vi "333D01.vi"() -> ()   [LabVIEW 2012]
uses:
  333D Queue Actions.ctl
  <vilib>/Analysis/4window.llb/windowTd.ctl
  <vilib>/sound2/lvsound2.llb/Sound Input Read (DBL).vi
  <vilib>/Analysis/5stat.llb/RMS (DBL).vi
  <vilib>/Analysis/0measdsp.llb/Scaled Time Domain Window (DBL).vi
  <vilib>/Analysis/NI_AALPro.lvlib
panel:
  out "333D01 Information":T1
  out "AvgCounts":u16 caption="/"
  in  "Average Counts":u16=10
  in  "Average":bool
  in  "Sample Rate (Hz)":dbl(ring)=8000.0 items=["8000 Hz"=8000.0, "11025 Hz"=11025.0, "16000 Hz"=16000.0, "22050 Hz"=22050.0, "32000 Hz"=32000.0, "44100 Hz"=44100.0, "48000 Hz"=48000.0]
  in  "Enable Cursor Reading":bool=TRUE
  in  "1st Cursor  to  Max Y":bool=TRUE caption="Harmonic Cursor\nwith 1st Cursor  to  Max Y"
  out "B: Sens (mV/g)":dbl caption="B:"
  out "A: Sens (mV/g)":dbl caption="A:"
  out "B: Overall (mV-rms)":dbl caption="B:" format="%#_4g"
  out "A: Overall (mV-rms)":dbl caption="A:" format="%#_4g"
  out "B: Overall (g-rms)":dbl caption="B:" format="%0.4f"
  out "A: Overall (g-rms)":dbl caption="A:" format="%0.4f"
  out "Cursors":string[][](table)
  in  "Enable Cursors":bool=TRUE
  in  "Window":T2=6 items=["Rectangle"=0, "Hanning"=1, "Hamming"=2, "Blackman-Harris"=3, "Exact Blackman"=4, "Blackman"=5, "Flat Top"=6, "4 Term B-Harris "=7, "7 Term B-Harris"=8, "Low Sidelobe"=9, "Blackman Nuttall"=11, "Triangle"=30, "Bartlett-Hanning"=31, "Bohman"=32, "Parzen"=33, "Welch"=34, "Kaiser"=60, "Dolph-Chebyshev"=61, "Gaussian"=62]
  in  "Aquire":bool=TRUE
  in  "Analyze":bool
  out "String":string
  in  "Queue Actions":T3
  out "B: Max (mV)":dbl
  out "A: Max (mV)":dbl
  in  "Sensitivity B (Counts / m/s^2)":i32=72139 caption="Chan B"
  in  "Sensitivity A (Counts / m/s^2)":i32=37426 caption="Chan A"
  out "Freq (Hz)":dbl
  out "B: Max (g peak)":dbl
  out "Spec":cluster{"Y":dbl[], "Y":dbl[]}[](graph)
  out "max index(es)":i32
  out "A: Max (g peak)":dbl
  out "Windowed":waveform(dbl)[](graph)
  out "data":waveform(dbl)[](array[waveform])
  out "Device Name":string
  in  "Device ID":u32
  out "Time":waveform(dbl)[](graph)
  in  "number of samples/ch":i32=4096
  in  "Quit":bool
  # "Overall (mV-rms):"
  # "Sensitivity (mV/g):"
  # "Overall (g-rms)"
  # "Acquisition Setup"
  # "Sensor Information"
  # "Sensitivity (Counts / m/s^2)"
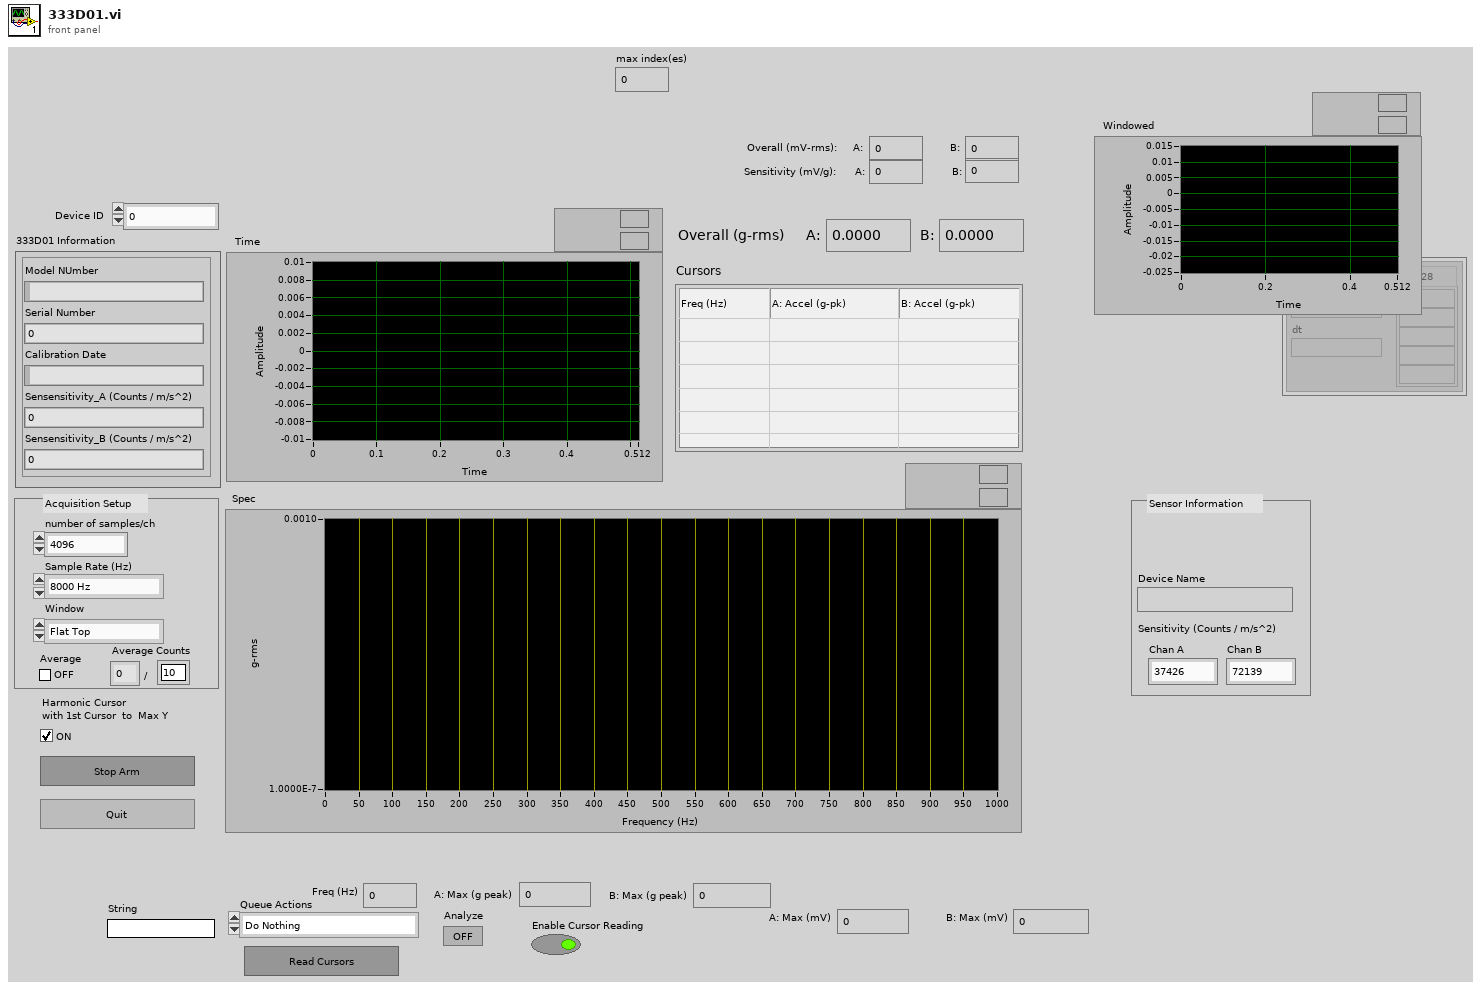
[diagram p1: front panel]
types:
  T1 = cluster{"Model NUmber":string, "Calibration Date":string, "Sensensitivity_A (Counts / m/s^2)":u64, "Sensensitivity_B (Counts / m/s^2)":u64, "Serial Number":u64}
  T2 = typedef "NI_AALPro.lvlib/windowTd.ctl" = u32
  T3 = typedef "333D Queue Actions.ctl" = enum16{"Do Nothing", "Initialize", "Process Data", "Process Cursors", "Pick Cursor", "Return"}
  T4 = cluster{"Model NUmber":string, "Calibration Date":string, "Sensensitivity_A":u64, "Sensensitivity_B":u64, "Serial Number":u64}
  T5 = cluster{"Sample Rate (Hz)":dbl, "Channels":i32, "Bits":i32}
  T6 = typedef "Sound Input Task ID.ctl" = u32
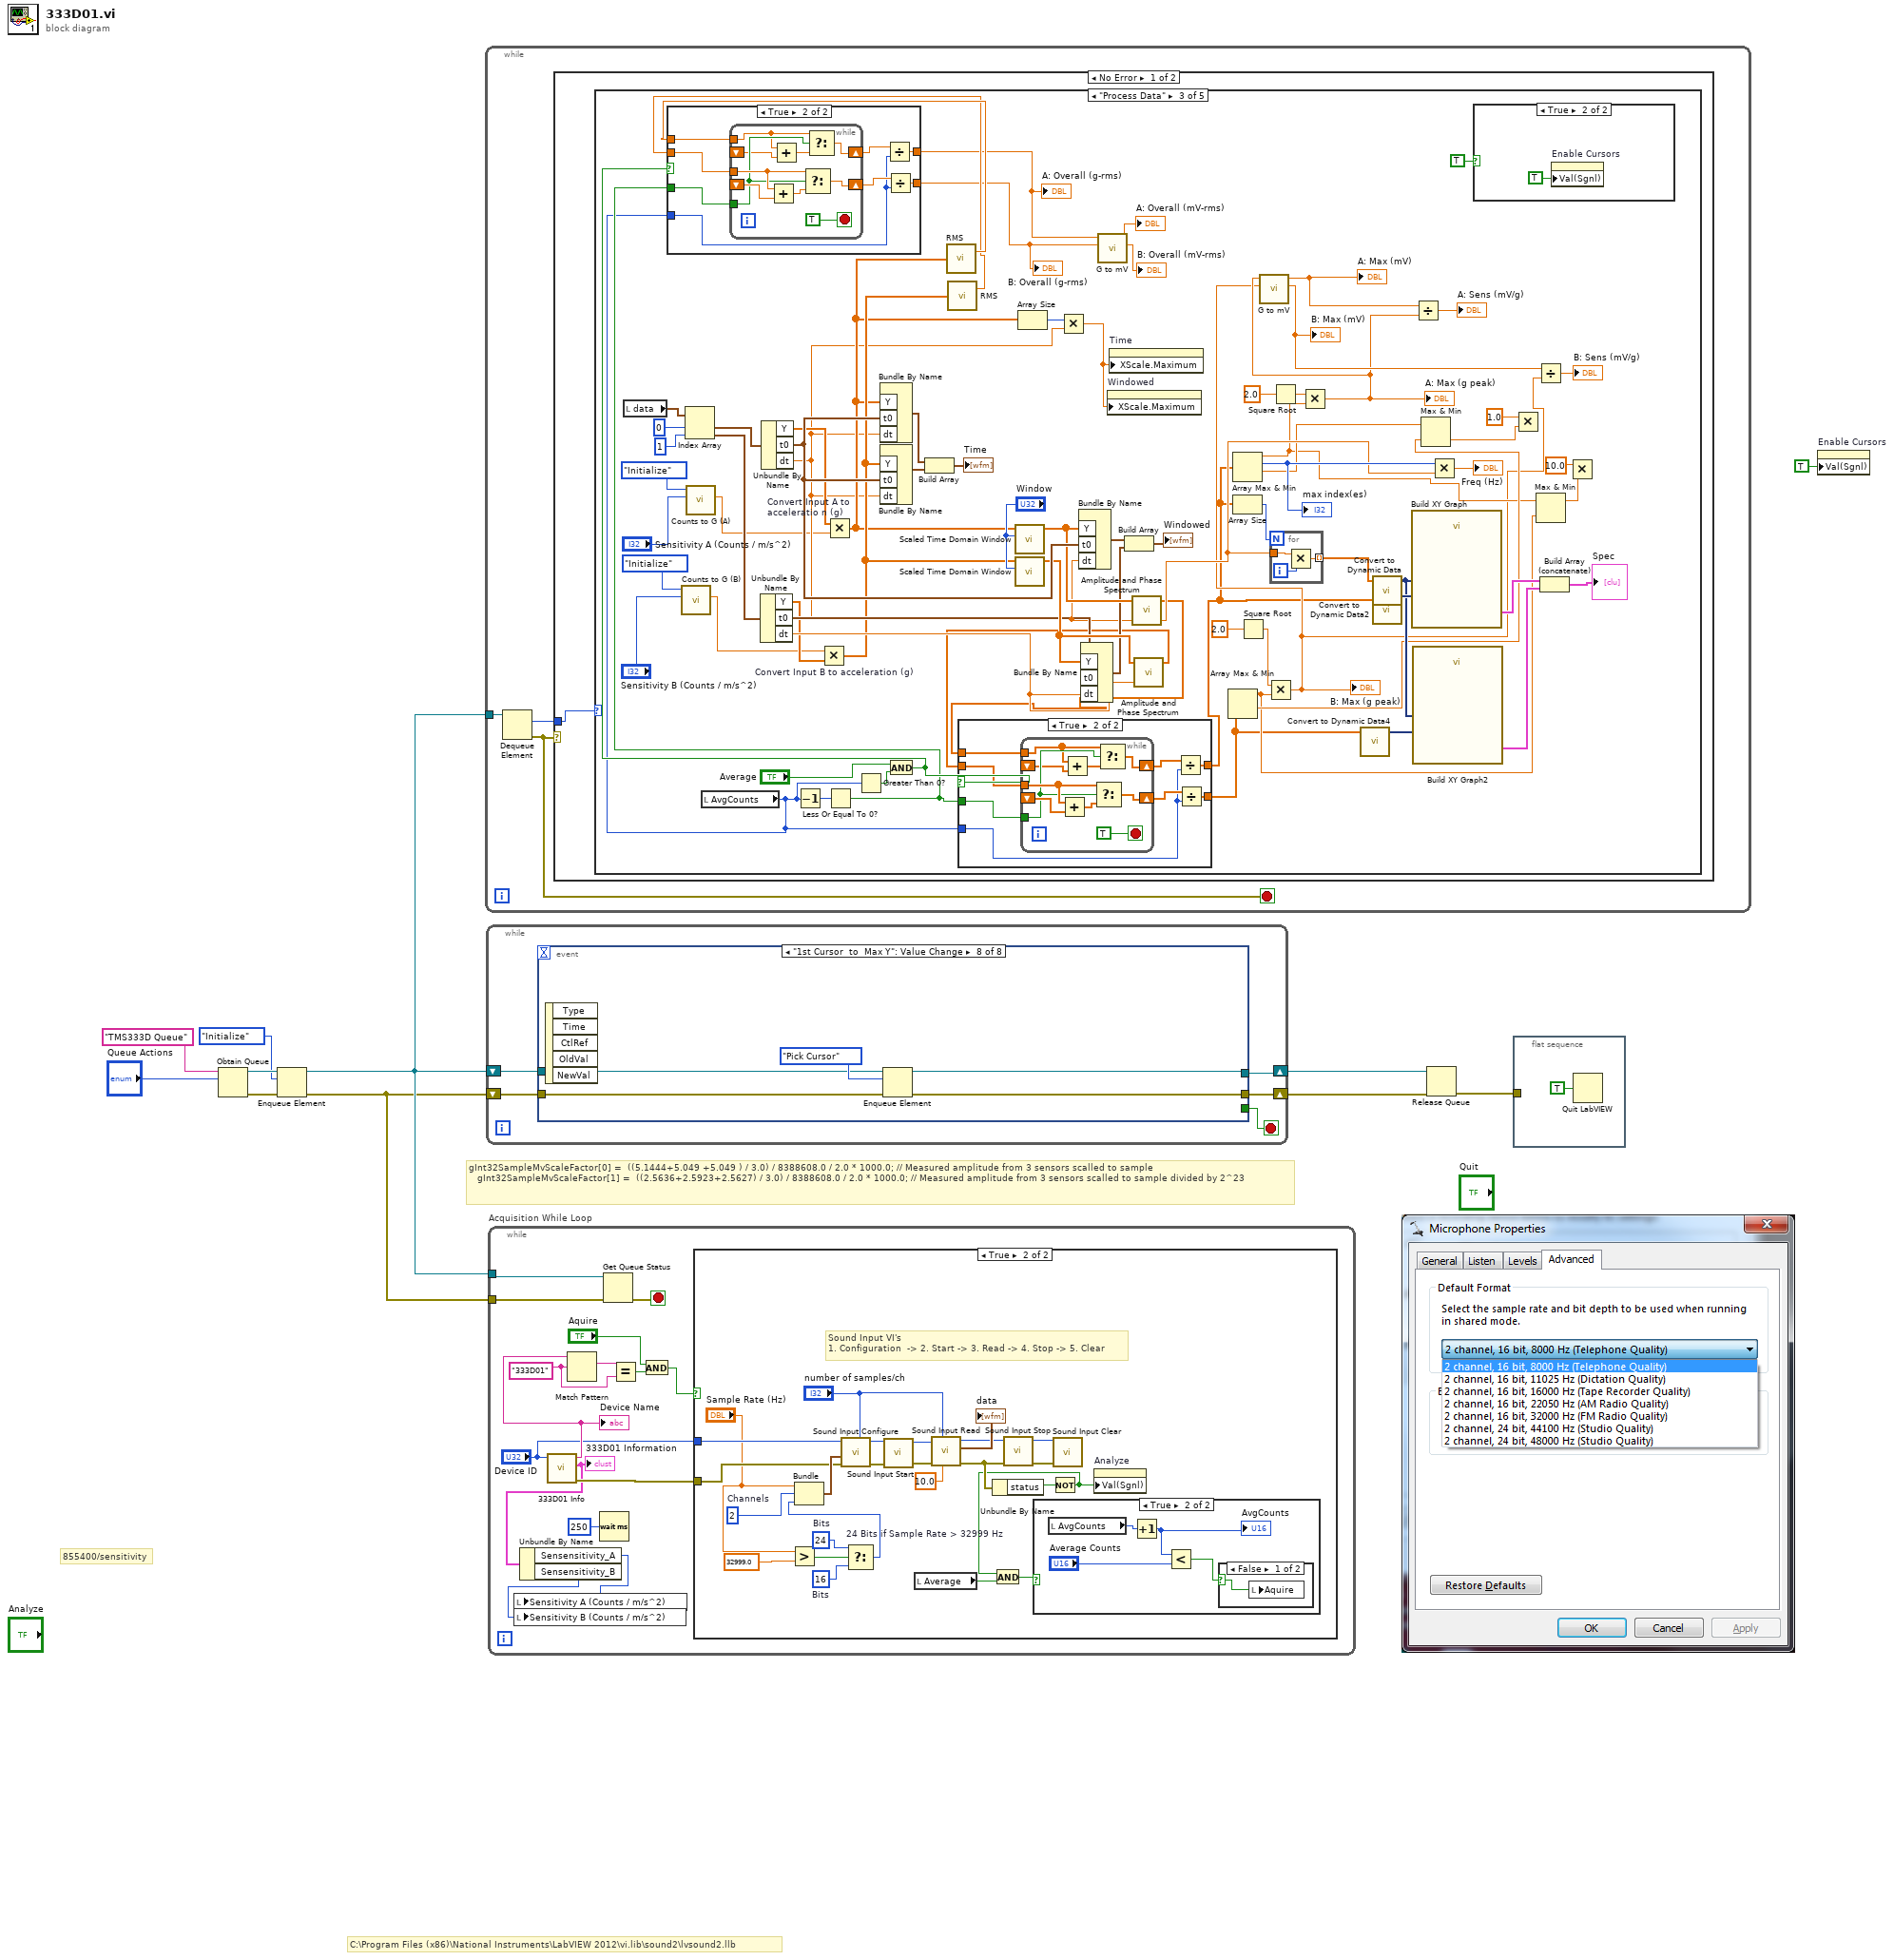
[diagram p0: block diagram]
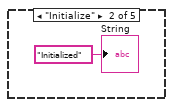
[diagram p6: hidden frame]
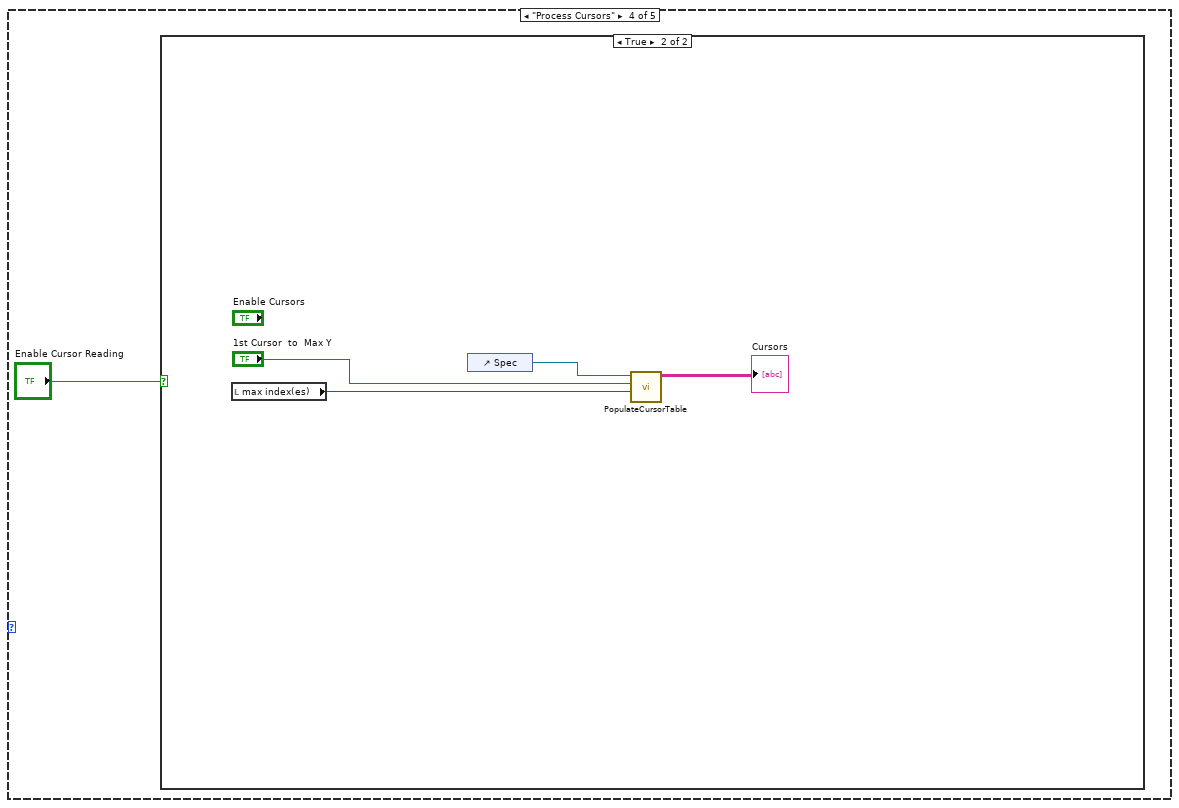
[diagram p10: hidden frame]
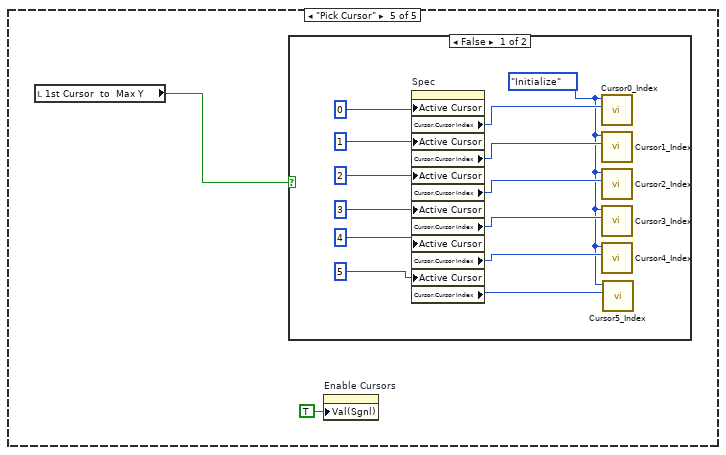
[diagram p12: hidden frame]
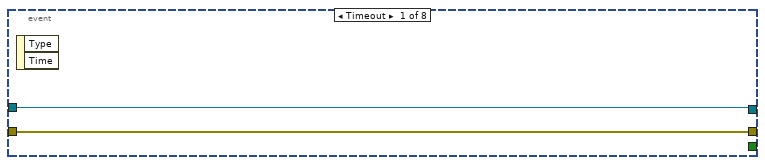
[diagram p15: hidden frame]
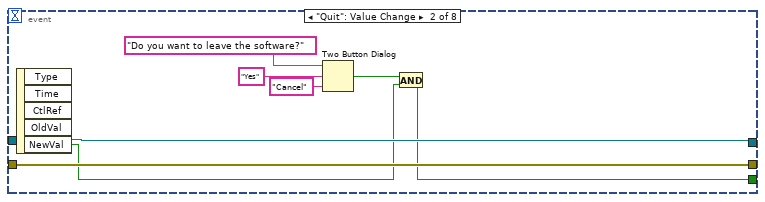
[diagram p16: hidden frame]
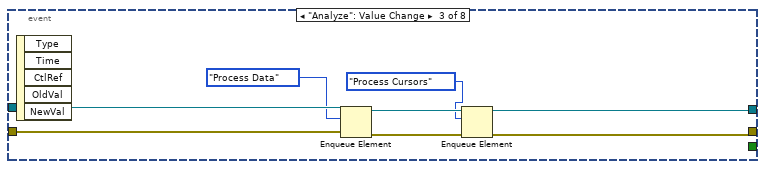
[diagram p17: hidden frame]
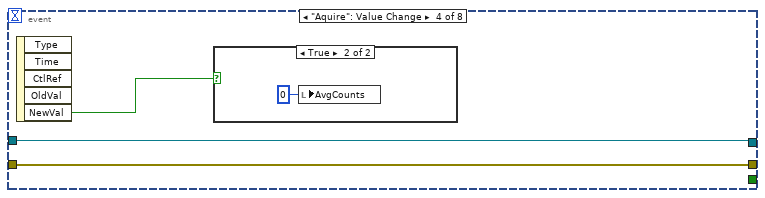
[diagram p18: hidden frame]
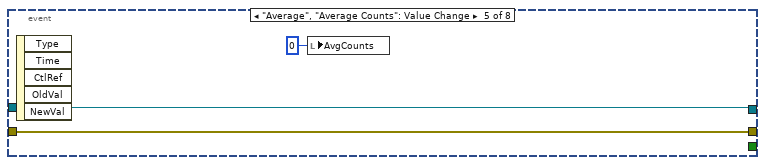
[diagram p20: hidden frame]
diagram:
  # "gInt32SampleMvScaleFactor[0] =  ((5.1444+5.049 +5.049 ) / 3.0) / 8388608.0 / 2.0 * 1000.0; // Measured amplitude from 3 sensors scalled to sample\n\t\t\tgInt32SampleMvScaleFactor[1] =  ((2.5636+2.5923+2.5627) / 3.0) / 8388608.0 / 2.0 * 1000.0; // Measured amplitude from 3 sensors scalled to sample divided by 2^23"
  # "855400/sensitivity"
  # "C:\\Program Files (x86)\\National Instruments\\LabVIEW 2012\\vi.lib\\sound2\\lvsound2.llb"
  n1 = Obtain Queue(name (unnamed)="TMS333D Queue", element data type="Queue Actions") -> (queue out=w9:refnum<queue>, error out=w8:errorcluster)  [unwired: 3 in, 1 out]
  n2 = Enqueue Element(queue=w9, element=333D_Queue_Actions."Initialize" ("Queue Actions"), error in (no error)=w8) -> (queue out=w4:refnum<queue>, error out=w3:errorcluster)  [unwired: 1 in, 1 out]
  n3 = while {
    tunnel: w4 -> [w14]
    stop <- w13 stop-if-true
    n4 = Dequeue Element(queue=w14) -> (element=w12:T3, error out=w13:errorcluster)  [unwired: 2 in, 2 out]
    n5 = case shown="No Error" w13 {
      tunnel: w12 -> [w15 _]
      frame No Error {
        n6 = case shown="\"Process Data\"" w15 {
          frame "Do Nothing", Default {
          }
          frame "Initialize" {
            "String" <- "Initialized" ("String")
          }
          frame "Process Data" {
            n7 = local read "data"() -> (w61:waveform(dbl)[])
            n8 = call "Counts to G (B).vi"("(Counts / m/s^2)"="Sensitivity B (Counts / m/s^2)", "Action"=enum16{"Initialize", "Read"}."Initialize") -> ("OutputB (g)"=w39:dbl)  [unwired: 8 in, 1 out]
            n9 = Index Array(array=w61, index #1=0 ("index"), index #2=1 ("index")) -> (element #1=w63:waveform(dbl), element #2=w66:waveform(dbl))
            n10 = call "Counts to G (A).vi"("(Counts / m/s^2)"="Sensitivity A (Counts / m/s^2)", "Action"=enum16{"Initialize", "Read"}."Initialize") -> ("Output (g)"=w41:dbl)  [unwired: 8 in, 1 out]
            n11 = local read "AvgCounts"() -> (w17:u16)
            n12 = Unbundle By Name(w66) -> ("Y"=w67:dbl[], "t0"=w68:timestamp, "dt"=w73:dbl)
            n13 = Unbundle By Name(w63) -> ("Y"=w89:dbl[], "t0"=w91:timestamp, "dt"=w48:dbl)
            n14 = Decrement(x=w17) -> (x-1=w30:u16)
            n15 = Multiply "Convert Input B to acceleration (g)"(x=w39, y=w67) -> (x*y=w54:dbl[])
            n16 = Multiply "Convert Input A to acceleratio n (g)"(x=w89, y=w41) -> (x*y=w50:dbl[])
            n17 = Less Or Equal To 0?(x=w30) -> (x <= 0?=w20:bool)
            n18 = Greater Than 0?(x=w17) -> (x > 0?=w18:bool)
            n19 = Bundle By Name("Y"=w50, "t0"=w91, "dt"=w48) -> (w88:waveform(dbl))  [unwired: 1 in]
            n20 = Bundle By Name("Y"=w54, "t0"=w91, "dt"=w48) -> (w92:waveform(dbl))  [unwired: 1 in]
            n21 = And(x="Average", y=w18) -> (x .and. y?=w21:bool)
            n22 = Build Array(w88, w92) -> (→"Time":waveform(dbl)[])
            n23 = call-poly <vilib>:"RMS.vi"("X"=w50) -> ("rms value"=w26:dbl)  [unwired: 1 out]
            n24 = call-poly <vilib>:"RMS.vi"("X"=w54) -> ("rms value"=w25:dbl)  [unwired: 1 out]
            n25 = case shown="True" w21 {
              tunnel: w25 -> [w94 w102]
              tunnel: w20 -> [_ w101]
              tunnel: w17 -> [_ w96]
              tunnel: [w94 w99] -> w22
              tunnel: w26 -> [w93 w98]
              tunnel: [w93 w95] -> w23
              frame False {
              }
              frame True {
                n26 = while {
                  shift-right: [w111] -> w100
                  shift-left: _ -> [w109]
                  tunnel: w102 -> [w110]
                  tunnel: w101 -> [w106]
                  tunnel: w98 -> [w105]
                  shift-right: [w107] -> w97
                  shift-left: _ -> [w104]
                  stop <- TRUE stop-if-true
                  n27 = Add(x=w110, y=w109) -> (x+y=w108:dbl)
                  n28 = Add(x=w105, y=w104) -> (x+y=w103:dbl)
                  n29 = Select(t=w110, s=w106, f=w108) -> (s? t:f=w111:dbl)
                  n30 = Select(t=w105, s=w106, f=w103) -> (s? t:f=w107:dbl)
                }
                n31 = Divide(x=w97, y=w96) -> (x/y=w95:dbl)
                n32 = Divide(x=w100, y=w96) -> (x/y=w99:dbl)
              }
            }
            "A: Overall (g-rms)" <- w23
            "B: Overall (g-rms)" <- w22
            n33 = call-poly <vilib>:"Scaled Time Domain Window.vi"("window"="Window", "X"=w50) -> ("Windowed X"=w71:dbl[])  [unwired: 7 in, 2 out]
            n34 = call-poly <vilib>:"Scaled Time Domain Window.vi"("window"="Window", "X"=w54) -> ("Windowed X"=w72:dbl[])  [unwired: 7 in, 2 out]
            n35 = Array Size(array=w50) -> (size(s)=w49:i32)
            n36 = Multiply(x=w49, y=w48) -> (x*y=w47:dbl)
            n37 = Bundle By Name("Y"=w71, "t0"=w91, "dt"=w48) -> (w64:waveform(dbl))  [unwired: 1 in]
            n38 = Bundle By Name("Y"=w72, "t0"=w68, "dt"=w73) -> (w70:waveform(dbl))  [unwired: 1 in]
            n39 = call "G to mV.vi"("Ain (g)"=w22, "Bin (g)"=w23) -> ("B out (mV)"=→"B: Overall (mV-rms)":dbl, "A out (mV)"=→"A: Overall (mV-rms)":dbl)  [unwired: 6 in]
            n40 = property on="Windowed" class="WFGraph (strict)"("XScale.Maximum"=w47) -> ()  [unwired: 2 in, 2 out]
            n41 = property on="Time" class="WFGraph (strict)"("XScale.Maximum"=w47) -> ()  [unwired: 2 in, 2 out]
            n42 = Build Array(w64, w70) -> (→"Windowed":waveform(dbl)[])
            n43 = call <vilib>:"Amplitude and Phase Spectrum.vi"("dt"=w48, "Signal (V)"=w71) -> ("df"=w81:dbl, "Amp Spectrum Mag (Vrms)"=w28:dbl[])  [unwired: 1 in, 1 out]
            n44 = call <vilib>:"Amplitude and Phase Spectrum.vi"("dt"=w73, "Signal (V)"=w72) -> ("Amp Spectrum Mag (Vrms)"=w31:dbl[])  [unwired: 1 in, 2 out]
            n45 = case shown="True" w21 {
              tunnel: w31 -> [w114 w122]
              tunnel: w20 -> [_ w121]
              tunnel: w17 -> [_ w116]
              tunnel: [w114 w119] -> w29
              tunnel: w28 -> [w113 w118]
              tunnel: [w113 w115] -> w27
              frame False {
              }
              frame True {
                n46 = while {
                  shift-right: [w131] -> w120
                  shift-left: _ -> [w129]
                  tunnel: w122 -> [w130]
                  tunnel: w121 -> [w126]
                  tunnel: w118 -> [w125]
                  shift-right: [w127] -> w117
                  shift-left: _ -> [w124]
                  stop <- TRUE stop-if-true
                  n47 = Add(x=w130, y=w129) -> (x+y=w128:dbl[])
                  n48 = Add(x=w125, y=w124) -> (x+y=w123:dbl[])
                  n49 = Select(t=w130, s=w126, f=w128) -> (s? t:f=w131:dbl[])
                  n50 = Select(t=w125, s=w126, f=w123) -> (s? t:f=w127:dbl[])
                }
                n51 = Divide(x=w117, y=w116) -> (x/y=w115:dbl[])
                n52 = Divide(x=w120, y=w116) -> (x/y=w119:dbl[])
              }
            }
            n53 = Array Max & Min(array=w29) -> (max value=w52:dbl, min value=w57:dbl)  [unwired: 2 out]
            n54 = Array Max & Min(array=w27) -> (max value=w53:dbl, max index (indices)=w82:i32, min value=w58:dbl)  [unwired: 1 out]
            "max index(es)" <- w82
            n55 = Array Size(array=w27) -> (size(s)=w74:i32)
            n56 = Square Root(x=2.0) -> (sqrt(x)=w87:dbl)
            n57 = Multiply(x=w87, y=w52) -> (x*y=w35:dbl)
            "B: Max (g peak)" <- w35
            n58 = for {
              N: w74 -> [_]
              tunnel: w81 -> [w135]
              tunnel: [w134] -> w76 mode=indexing
              i -> [w136]
              n59 = Multiply(x=w135, y=w136) -> (x*y=w134:dbl)
            }
            n60 = Square Root(x=2.0) -> (sqrt(x)=w84:dbl)
            n61 = Multiply(x=w84, y=w53) -> (x*y=w36:dbl)
            "A: Max (g peak)" <- w36
            n62 = call "G to mV.vi"("Ain (g)"=w35, "Bin (g)"=w36) -> ("B out (mV)"=w45:dbl, "A out (mV)"=w46:dbl)  [unwired: 6 in]
            "A: Max (mV)" <- w46
            "B: Max (mV)" <- w45
            n63 = call "Convert to Dynamic Data4"("Array"=w29) -> ("Dynamic Data Type"=w75:dynamicdata)  [unwired: 3 in]
            n64 = call "Convert to Dynamic Data"("Array"=w76) -> ("Dynamic Data Type"=w59:dynamicdata)  [unwired: 3 in]
            n65 = call "Convert to Dynamic Data2"("Array"=w27) -> ("Dynamic Data Type"=w77:dynamicdata)  [unwired: 3 in]
            n66 = call "Build XY Graph"("Y Input"=w77, "X Input"=w59) -> ("XY Graph"=w78:cluster{"Y":dbl[], "Y":dbl[]}[])  [unwired: 3 in, 6 out]
            n67 = call "Build XY Graph2"("Y Input"=w75, "X Input"=w59) -> ("XY Graph"=w79:cluster{"Y":dbl[], "Y":dbl[]}[])  [unwired: 3 in, 6 out]
            n68 = Divide(x=w46, y=w36) -> (x/y=→"A: Sens (mV/g)":dbl)
            n69 = Max & Min(x=w58, y=w57) -> (min(x,y)=w56:dbl)  [unwired: 1 out]
            n70 = Multiply(x=w82, y=w81) -> (x*y=→"Freq (Hz)":dbl)
            n71 = case shown="True" TRUE {
              frame False {
              }
              frame True {
                n72 = property on="Enable Cursors" class="Bool (strict)"("Val(Sgnl)"=TRUE ("Value (Signaling)")) -> ()  [unwired: 2 in, 2 out]
              }
            }
            n73 = Multiply(x=1.0, y=w56) -> ()  [unwired: 1 out]
            n74 = Divide(x=w45, y=w35) -> (x/y=→"B: Sens (mV/g)":dbl)
            n75 = Max & Min(x=w53, y=w52) -> (max(x,y)=w51:dbl)  [unwired: 1 out]
            n76 = Build Array (concatenate)(w78, w79) -> (→"Spec":cluster{"Y":dbl[], "Y":dbl[]}[])
            n77 = Multiply(x=10.0, y=w51) -> ()  [unwired: 1 out]
          }
          frame "Process Cursors" {
            n78 = case shown="True" "Enable Cursor Reading" {
              frame False {
              }
              frame True {
                n79 = local read "max index(es)"() -> (w140:i32)
                n80 = control-ref of="Spec"() -> (w138:refnum<vi>)
                n81 = call "PopulateCursorTable.vi"("max index(es)"=w140, "1st Cursor  to  Max Y"="1st Cursor  to  Max Y", "XYGraph in"=w138) -> ("Array"=→"Cursors":string[][])  [unwired: 8 in]
              }
            }
          }
          frame "Pick Cursor" {
            n82 = local read "1st Cursor  to  Max Y"() -> (w143:bool)
            n83 = case shown="False" w143 {
              frame False {
                w145 = enum16{"Initialize", "Read"}."Initialize" ("Action")
                n84 = property on="Spec" class="XYGraph (strict)"("Active Cursor"=u32 0, "Active Cursor"=1 ("Cursor.Cursor Index"), "Active Cursor"=u32 2, "Active Cursor"=u32 3, "Active Cursor"=u32 4, "Active Cursor"=u32 5) -> ("Cursor.Cursor Index"=w151:i32, "Cursor.Cursor Index"=w150:i32, "Cursor.Cursor Index"=w149:i32, "Cursor.Cursor Index"=w148:i32, "Cursor.Cursor Index"=w147:i32, "Cursor.Cursor Index"=w144:i32)  [unwired: 2 in, 2 out]
                n85 = call "Cursor0_Index.vi"("Input"=w151, "Action"=w145) -> ()  [unwired: 8 in, 2 out]
                n86 = call "Cursor1_Index.vi"("Input"=w150, "Action"=w145) -> ()  [unwired: 8 in, 2 out]
                n87 = call "Cursor2_Index.vi"("Input"=w149, "Action"=w145) -> ()  [unwired: 8 in, 2 out]
                n88 = call "Cursor3_Index.vi"("Input"=w148, "Action"=w145) -> ()  [unwired: 8 in, 2 out]
                n89 = call "Cursor4_Index.vi"("Input"=w147, "Action"=w145) -> ()  [unwired: 8 in, 2 out]
                n90 = call "Cursor5_Index.vi"("Input"=w144, "Action"=w145) -> ()  [unwired: 8 in, 2 out]
              }
              frame True {
              }
            }
            n91 = property on="Enable Cursors" class="Bool (strict)"("Val(Sgnl)"=TRUE ("Value (Signaling)")) -> ()  [unwired: 2 in, 2 out]
          }
        }
      }
      frame Error {
      }
    }
  }
  n92 = while {
    shift-right: [w159] -> w6
    shift-left: w4 -> [w161]
    shift-right: [w158] -> w5
    shift-left: w3 -> [w160]
    stop <- w157 stop-if-true
    n93 = event shown="[7] \"1st Cursor  to  Max Y\": Value Change" {
      selector: _ -> [_ _ _ _ _ _ _ _]
      dyn-events: _ -> [_ _ _ _ _ _ _ _]
      timeout: _ -> [_ _ _ _ _ _ _ _]
      tunnel: [w163 w171 w175 w182 w186 w190 w200 w205] -> w159
      tunnel: w161 -> [w163 w171 w179 w182 w186 w191 w202 w207]
      tunnel: w160 -> [w162 w170 w178 w181 w185 w189 w201 w206]
      tunnel: [w162 w170 w173 w181 w185 w188 w199 w204] -> w158
      tunnel: [_ w164 _ _ _ _ _ _] -> w157
      event Timeout {
        n94 = event-data() -> ()  [unwired: 1 in, 2 out]
      }
      event "Quit": Value Change {
        n95 = event-data() -> ("NewVal"=w165:bool)  [unwired: 1 in, 4 out]
        n96 = Two Button Dialog(message="Do you want to leave the software?", 1:"Cancel" ("F button name (\"Cancel\")"), 2:"Yes" ("T button name (\"OK\")")) -> (T button?=w166:bool)
        n97 = And(x=w166, y=w165) -> (x .and. y?=w164:bool)
      }
      event "Analyze": Value Change {
        n98 = event-data() -> ()  [unwired: 1 in, 5 out]
        n99 = Enqueue Element(queue=w179, element=333D_Queue_Actions."Process Data", error in (no error)=w178) -> (queue out=w176:refnum<queue>, error out=w174:errorcluster)  [unwired: 1 in, 1 out]
        n100 = Enqueue Element(queue=w176, element=333D_Queue_Actions."Process Cursors", error in (no error)=w174) -> (queue out=w175:refnum<queue>, error out=w173:errorcluster)  [unwired: 1 in, 1 out]
      }
      event "Aquire": Value Change {
        n101 = event-data() -> ("NewVal"=w180:bool)  [unwired: 1 in, 4 out]
        n102 = case shown="True" w180 {
          frame False {
          }
          frame True {
            n103 = local write "AvgCounts"(u16 0 ("AvgCounts")) -> ()
          }
        }
      }
      event "Average", "Average Counts": Value Change {
        n104 = event-data() -> ()  [unwired: 1 in, 5 out]
        n105 = local write "AvgCounts"(u16 0 ("AvgCounts")) -> ()
      }
      event "Enable Cursors": Value Change {
        n106 = event-data() -> ()  [unwired: 1 in, 5 out]
        n107 = case shown="True" TRUE {
          tunnel: w191 -> [w193 w198]
          tunnel: [w193 w197] -> w190
          tunnel: w189 -> [w192 w196]
          tunnel: [w192 w195] -> w188
          frame False {
          }
          frame True {
            n108 = Enqueue Element(queue=w198, element=333D_Queue_Actions."Process Cursors", error in (no error)=w196) -> (queue out=w197:refnum<queue>, error out=w195:errorcluster)  [unwired: 1 in, 1 out]
          }
        }
      }
      event "Spec": Cursor Move; "Spec": Cursor Grab; "Spec": Cursor Release {
        n109 = event-data() -> ()  [unwired: 1 in, 6 out]
        n110 = Enqueue Element(queue=w202, element=333D_Queue_Actions."Pick Cursor", error in (no error)=w201) -> (queue out=w200:refnum<queue>, error out=w199:errorcluster)  [unwired: 1 in, 1 out]
      }
      event "1st Cursor  to  Max Y": Value Change {
        n111 = event-data() -> ()  [unwired: 1 in, 5 out]
        n112 = Enqueue Element(queue=w207, element=333D_Queue_Actions."Pick Cursor", error in (no error)=w206) -> (queue out=w205:refnum<queue>, error out=w204:errorcluster)  [unwired: 1 in, 1 out]
      }
    }
  }
  n113 = while "Acquisition While Loop" {
    tunnel: w4 -> [w218]
    tunnel: w3 -> [w217]
    stop <- w216 stop-if-true
    w222 = "333D01" ("regular expression")
    n114 = call "333D01 Info.vi"("deviceID"="Device ID") -> ("error out"=w213:errorcluster, "333D01 Info"=w211:T4, "Device Name"=w215:string)  [unwired: 8 in]
    "Device Name" <- w215
    "333D01 Information" <- w211
    n115 = Unbundle By Name(w211) -> ("Sensensitivity_A"=w210:u64, "Sensensitivity_B"=w209:u64)
    n116 = local write "Sensitivity A (Counts / m/s^2)"(w210) -> ()
    n117 = local write "Sensitivity B (Counts / m/s^2)"(w209) -> ()
    n118 = Match Pattern(string=w215, regular expression=w222) -> (match substring=w223:string)  [unwired: 1 in, 3 out]
    n119 = Wait (ms)(milliseconds to wait=u32 250) -> ()  [unwired: 1 out]
    n120 = Get Queue Status(queue=w218, error in (no error)=w217) -> (error out=w216:errorcluster)  [unwired: 1 in, 7 out]
    n121 = Equal?(x=w223, y=w222) -> (x = y?=w221:bool)
    n122 = And(x="Aquire", y=w221) -> (x .and. y?=w220:bool)
    n123 = case shown="True" w220 {
      tunnel: "Device ID" -> [_ w234]
      tunnel: w213 -> [_ w233]
      frame False {
      }
      frame True {
        w230 = 16  # Bits
        w229 = 24  # Bits
        w242 = 2  # Channels
        # "Sound Input VI's\n1. Configuration  -> 2. Start -> 3. Read -> 4. Stop -> 5. Clear"
        n124 = Greater?(x="Sample Rate (Hz)", y=32999.0) -> (0:w228:bool)
        n125 = Select "24 Bits if Sample Rate > 32999 Hz"(t=w229, s=w228, f=w230) -> (s? t:f=w227:i32)
        n126 = Bundle("Sample Rate (Hz)"="Sample Rate (Hz)", "Channels"=w242, "Bits"=w227) -> (w243:T5)  [unwired: 1 in]
        n127 = call <vilib>:"Sound Input Configure.vi"("number of samples/ch"="number of samples/ch", "error in (no error)"=w233, "sound format"=w243, "device ID"=w234) -> ("error out"=w248:errorcluster, "task ID"=w247:T6)  [unwired: 6 in]
        n128 = call <vilib>:"Sound Input Start.vi"("error in (no error)"=w248, "task ID"=w247) -> ("error out"=w244:errorcluster, "task ID out"=w246:T6)  [unwired: 8 in]
        n129 = local read "Average"() -> (w226:bool)
        n130 = call-poly <vilib>:"Sound Input Read.vi"("timeout (sec)"=10.0, "number of samples/ch"="number of samples/ch", "error in (no error)"=w244, "task ID"=w246) -> ("error out"=w235:errorcluster, "data"=→"data":waveform(dbl)[], "task ID out"=w237:T6)  [unwired: 5 in]
        n131 = Unbundle By Name(w235) -> ("status"=w236:bool)
        n132 = call <vilib>:"Sound Input Stop.vi"("error in (no error)"=w235, "task ID"=w237) -> ("error out"=w239:errorcluster, "task ID out"=w238:T6)  [unwired: 8 in]
        n133 = Not(x=w236) -> (.not. x?=w225:bool)
        n134 = And(x=w225, y=w226) -> (x .and. y?=w224:bool)
        n135 = case shown="True" w224 {
          frame False {
          }
          frame True {
            n136 = local read "AvgCounts"() -> (w252:u16)
            n137 = Increment(x=w252) -> (x+1=w250:u16)
            "AvgCounts" <- w250
            n138 = Less?(x=w250, y="Average Counts") -> (x < y?=w249:bool)
            n139 = case shown="False" w249 {
              selector: w249 -> [w253 _]
              frame False {
                n140 = local write "Aquire"(w253) -> ()
              }
              frame True {
              }
            }
          }
        }
        n141 = call <vilib>:"Sound Input Clear.vi"("error in (no error)"=w239, "task ID"=w238) -> ()  [unwired: 9 in, 1 out]
        n142 = property on="Analyze" class="Bool (strict)"("Val(Sgnl)"=w225) -> ()  [unwired: 2 in, 2 out]
      }
    }
  }
  n143 = Release Queue(queue=w6, error in (no error)=w5) -> (error out=w2:errorcluster)  [unwired: 1 in, 2 out]
  n144 = flat-sequence {
    tunnel: w2 -> [_]
    frame #0 {
      n145 = Quit LabVIEW(quit? (T)=TRUE) -> ()
    }
  }
  n146 = property on="Enable Cursors" class="Bool (strict)"("Val(Sgnl)"=TRUE ("Value (Signaling)")) -> ()  [unwired: 2 in, 2 out]
